vi "UMLEditor Main.vi"(1 "StartProject":string, 3 "StartTarget":string) -> ()   [LabVIEW 2012]
doc: "Main Open UML Modeller VI"
uses:
  <resource>/Framework/Providers/Open_GDS/UML/UMLEditor/UMLEditor ClassToolButtons.ctl
  <resource>/Framework/Providers/Open_GDS/UML/UMLEditor/UMLEditor SequenceToolButtons.ctl
  <resource>/Framework/Providers/Open_GDS/UML/UMLEditor/UMLEditor UseCaseToolButtons.ctl
  <resource>/Framework/Providers/Open_GDS/UML/UMLEditor/UMLEditor StateToolButtons.ctl
  <resource>/Framework/Providers/Open_GDS/UML/UMLEditor/UMLEditor statesType.ctl
  <resource>/Framework/Providers/Open_GDS/UML/UMLEditor/UMLEditor LocalVariablesType.ctl
  <resource>/Framework/Providers/Open_GDS/UML/Graphics_class/Graphics.lvclass
  <resource>/Framework/Providers/Open_GDS/UML/Grid_class/Grid.lvclass
  <resource>/Framework/Providers/Open_GDS/UML/UMLEditor/UMLEditor tooltype.ctl
  <resource>/Framework/Providers/Open_GDS/UML/UMLEditor/UMLEditor toolsType.ctl
  <resource>/Framework/Providers/Open_GDS/UML/Graph_class/private/diagramType.ctl
  <resource>/Framework/Providers/Open_GDS/UML/Graph_class/Graph.lvclass
  <resource>/Framework/Providers/Open_GDS/UML/General/Point/Point Point2D.ctl
  <resource>/Framework/Providers/Open_GDS/UML/General/Rectangle/Rectangle Rectangle2D.ctl
  <resource>/Framework/Providers/Open_GDS/UML/AbstractEdge_class/AbstractEdge.lvclass
  <resource>/Framework/Providers/Open_GDS/UML/UMLEditor/UMLEditor ExportType.ctl
  <resource>/Framework/Providers/Open_GDS/UML/UMLEditor/UMLEditor FlattenCommandType.ctl
  <resource>/Framework/Providers/Open_GDS/UML/UMLEditor/UMLEditor ExecuteCommandType.ctl
  <resource>/Framework/Providers/Open_GDS/UML/ContextHelp/ContextHelp_EventType.ctl
  <resource>/Framework/Providers/Open_GDS/UML/AbstractNode_class/AbstractNode.lvclass
  <resource>/Framework/Providers/Open_GDS/UML/UmlEditor_class/EventData.ctl
  <resource>/Framework/Providers/Open_GDS/UML/UMLEditor/UMLEditor_HotSpotData.ctl
  <resource>/Framework/Providers/Open_GDS/UML/UMLEditor/UMLEditor_HotSpotType.ctl
  <resource>/Framework/Providers/Open_GDS/UML/UMLEditor/UMLEditor_Cursortype.ctl
  <resource>/Framework/Providers/Open_GDS/UML/UMLEditor/UMLEditor MenuActionType.ctl
  <resource>/Framework/Providers/Open_GDS/UML/Graphics_class/LvFontType.ctl
  <resource>/Framework/Providers/Open_GDS/UML/UMLEditor/UMLEditor ToolButtonsAction.ctl
  <resource>/Framework/Providers/Open_GDS/UML/Graphics_class/FontType.ctl
  <resource>/Framework/Providers/Open_GDS/UML/UMLEditor/UMLEditor BusyDialogAction.ctl
  <resource>/Framework/Providers/Open_GDS/UML/UMLEditor/UMLEditor_StoredPathes.ctl
  <resource>/Framework/Providers/Open_GDS/ClassProviders/Common/File/File_StoredPathesActions.ctl
  <resource>/Framework/Providers/Open_GDS/UML/GeneralPathEdge_class/GeneralPathEdge.lvclass
  <vilib>/event_ctls.llb/eventvkey.ctl
  <resource>/Framework/Providers/Open_GDS/UML/ContextHelp/ContextHelp_HelpTexts.ctl
  <resource>/Framework/Providers/Open_GDS/UML/Graph_class/SaveTypes.ctl
  <resource>/Framework/Providers/Open_GDS/UML/ClassNode_class/ClassNode.lvclass
  <resource>/Framework/Providers/Open_GDS/UML/StateDiagramGraph_class/StateDiagramGraph.lvclass
  <resource>/Framework/Providers/Open_GDS/UML/ClassNode_class/ExternalSetTypes.ctl
  <resource>/Framework/Providers/Open_GDS/UML/StateDiagramGraph_class/private/StateDiagramData.ctl
  <resource>/Framework/Providers/Open_GDS/UML/StateDiagramGraph_class/private/ViPathShowOption.ctl
  <resource>/Framework/Providers/Open_GDS/UML/UMLEditor/UMLEditor ClipBoardActionType.ctl
  <resource>/Framework/Providers/Open_GDS/UML/RectangularNode_class/RectangularNode.lvclass
  <resource>/Framework/Providers/Open_GDS/UML/ReversedEngineering/private/ReversedEngineering SyncUmlFromCodeActions.ctl
  <resource>/Framework/Providers/Open_GDS/ClassProviders/Provider_BaseClassInterface/ClassReader_class/ClassReader.lvclass
  <resource>/Framework/Providers/Open_GDS/ClassProviders/Common/CommonVIs/CommonVIs_StereoType.ctl
  <vilib>/Utility/cursorutil.llb/Set Cursor (Icon Pict).vi
  <vilib>/Utility/cursorutil.llb/Set Cursor (Cursor ID).vi
  Instance           2 22Saved   UMLEditor Main .vi
  Instance           1 22Saved   UMLEditor Main .vi
  <resource>/Framework/Providers/Open_GDS/UML/ClassDiagramGraph_class/ClassDiagramGraph.lvclass
  <resource>/Framework/Providers/Open_GDS/UML/SequenceDiagramGraph_class/SequenceDiagramGraph.lvclass
  <resource>/Framework/Providers/Open_GDS/UML/UseCaseDiagramGraph_class/UseCaseDiagramGraph.lvclass
  <resource>/Framework/Providers/Open_GDS/UML/UmlEditor_class/UmlEditor.lvclass
panel:
  out "SearchString":string caption="Search"
  in  "open":bool
  in  "close":bool
  in  "Diagram":u16(ring) items=["State diagram: State1.uml *"]
  out "toolTab":enum32{"Class", "Sequence", "UseCase", "State"}(tab)
  in  "classDiagramTools":T1={"select"=TRUE, "class"=FALSE, "interface"=FALSE, "package"=FALSE, "dependancy"=FALSE, "inheritance"=FALSE, "interfaceImp"=FALSE, "association"=FALSE, "aggregetion"=FALSE, "compAggregetion"=FALSE, "note"=FALSE, "noteConnect"=FALSE}
  in  "sequenceDiagramTools":T2={"select"=TRUE, "Object"=FALSE, "ActionBar"=FALSE, "Call"=FALSE, "note"=FALSE, "noteConnect"=FALSE}
  in  "usecaseDiagramTools":T3={"select"=TRUE, "System"=FALSE, "Actor"=FALSE, "UseCase"=FALSE, "Association"=FALSE, "Generalisation"=FALSE, "Includes"=FALSE, "Extends"=FALSE, "Note"=FALSE, "noteConnect"=FALSE}
  in  "stateDiagramTools":T4={"select"=TRUE, "State"=FALSE, "InitialState"=FALSE, "FinalState"=FALSE, "choice"=FALSE, "StateTransation"=FALSE, "note"=FALSE, "noteConnect"=FALSE}
  out "ProductPicture":picture
  out "Time":i32=21
  out "PictureMenuEvent":string
  out "RevHistory":bool
  in  "Help":bool
  in  "DragAndDropPath":path
  in  "ClassAggregationDialog":T5
  out "Picture":picture
  out "error out":errorcluster
  in  "Project":u16(ring) items=["Open_GDS.lvproj"]
  in  "Help":bool=TRUE
  in  "Case Constant\n(See Context Help) 2":bool
  in  "Target":u16(ring) items=["My Computer"]
  out "StatusBar":string
  in  "Sync":bool
  # "Class aggregation"
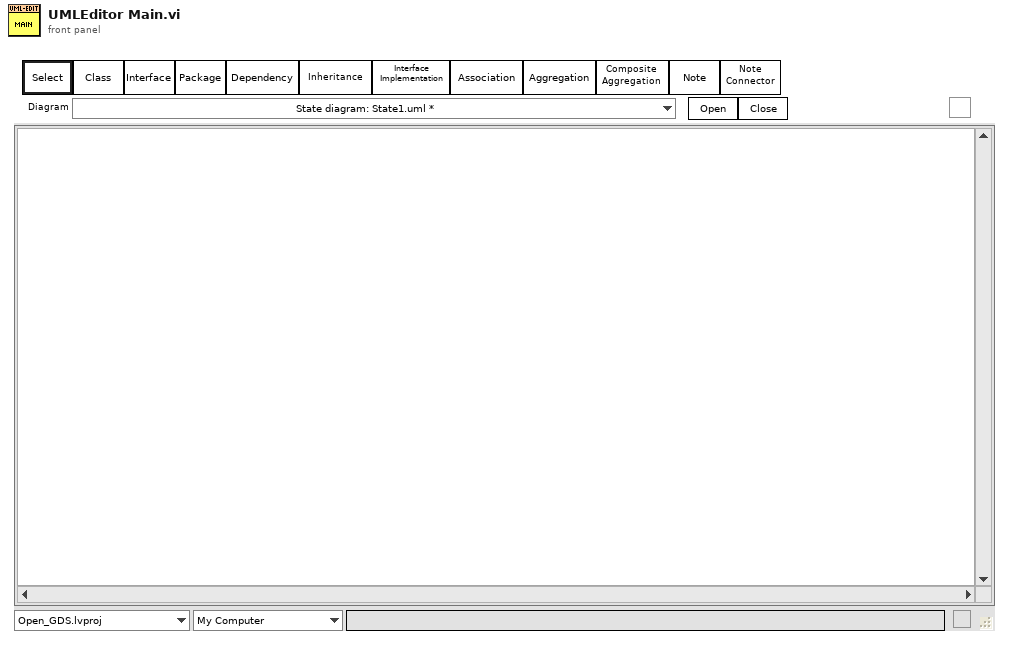
[diagram p1: front panel]
types:
  T1 = typedef "UMLEditor ClassToolButtons.ctl" = cluster{"select":bool, "class":bool, "interface":bool, "package":bool, "dependancy":bool, "inheritance":bool, "interfaceImp":bool, "association":bool, "aggregetion":bool, "compAggregetion":bool, "note":bool, "noteConnect":bool}
  T2 = typedef "UMLEditor SequenceToolButtons.ctl" = cluster{"select":bool, "Object":bool, "ActionBar":bool, "Call":bool, "note":bool, "noteConnect":bool}
  T3 = typedef "UMLEditor UseCaseToolButtons.ctl" = cluster{"select":bool, "System":bool, "Actor":bool, "UseCase":bool, "Association":bool, "Generalisation":bool, "Includes":bool, "Extends":bool, "Note":bool, "noteConnect":bool}
  T4 = typedef "UMLEditor StateToolButtons.ctl" = cluster{"select":bool, "State":bool, "InitialState":bool, "FinalState":bool, "choice":bool, "StateTransation":bool, "note":bool, "noteConnect":bool}
  T5 = cluster{"AddAttribute":bool, "Don'tAddAttribute":bool, "Close":bool, "Text":string}
  T6 = typedef "UMLEditor_Cursortype.ctl" = enum16{"NS", "WE", "NESW", "NWSE"}
  T7 = typedef "UMLEditor LocalVariablesType.ctl" = cluster{"state":T8, "graphics":refnum<class "Graphics.lvclass">, "grid":refnum<class "Grid.lvclass">, "toolType":T9, "tool":T10, "diagramIndex":i32, "diagrams":cluster{"name":string, "diagramType":T11, "unsaved":bool, "graph":refnum<class "Graph.lvclass">, "saveDir":path}[], "zoom":dbl, "hideGrid":bool, "lastMousePoint":T12, "rubberBandStart":T12, "dragStartPoint":T12, "dragStartBounds":T13, "gridColor":u32, "gridSize":dbl, "CONNECT_THRESHOLD":i32, "selcted":T9, "selectedEdge":refnum<class "AbstractEdge.lvclass">, "butDwn":bool, "lastPress":u32, "modified":bool, "offset":T12, "menu":refnum<k9>, "file":path, "saveAs":bool, "newSelected":bool, "exportype":T14, "quit":bool, "revHistory":cluster{"rev":string, "text":string}[], "FlattenCommandSettings":T15, "PopUpMessageEvent":T17, "ResizePanelInProgress":bool, "NodesBounds":T13, "ToolHelp":bool, "ViRef":refnum<vi>, "FP_CtrlEnterEvents":refnum<event-registration>, "SelectedNodes":refnum<class "AbstractNode.lvclass">[], "mouse":refnum<k1>, "RevPlugInPath":path, "Event":refnum<event-registration>, "Action":string, "KeyPressTime":u32, "Cursors":refnum<k1>[], "ObjectHotspots":T18[], "HotSpotCursor":bool, "HotSpotFunction":T19, "Don'tDeleteChildren":bool, "ShiftDown":bool, "CtrlDown":bool, "HotSpotNode":refnum<class "AbstractNode.lvclass">, "Sync":bool, "SyncTime":u32, "ForceSyncNow":bool, "LastSync":timestamp, "XMI_Import":bool}
  T8 = typedef "UMLEditor statesType.ctl" = enum16{"Idle", "CheckLicense", "revHistory", "Init", "Init2", "EditSelected", "RemoveSelected", "PaintComponent", "ChangeZoom", "ChangeGridSize", "Open", "Close", "Save", "ExportPicture", "Export", "Repaint", "Error", "Exit", "QUIT", "CreateScript", "ExecuteScript", "ClassReversedEngineering", "PlugInReverseEngineering", "StateReversedEngineering", "AutoPlace", "ExecuteCommand", "OpenClass", "SyncAll", "StraightenAssociation", "Copy", "Paste", "AddNodeFromProjectTree", "AddNodeFromProjectTree+SyncAll", "PanAndRepaint", "Init3", "CopyPaste", "ApplyDesignPattern", "AnalyseViInStateDiagram", "AutoSync"}
  T9 = typedef "UMLEditor tooltype.ctl" = enum16{"None", "Node", "Edge"}
  T10 = typedef "UMLEditor toolsType.ctl" = enum16{"CD_Select", "CD_Class", "CD_Interface", "CD_Package", "CD_Note", "CD_Dependency", "CD_Inheritance", "CD_InterfaceImp", "CD_Association", "CD_Aggregation", "CD_Composite", "CD_NoteConn", "SQD_Select", "SQD_Object", "SQD_ActionBar", "SQD_Note", "SQD_Call", "SQD_NoteConn", "UD_Select", "UD_System", "UD_Actor", "UD_UseCase", "UD_Note", "UD_Assoiciation", "UD_Generalization", "UD_GeneralizationIncludes", "UD_GeneralizationExtends", "UD_Realization", "UD_Relationship", "UD_NoteEdge", "STD_Select", "STD_State", "STD_InitailState", "STD_FinalState", "STD_ChoiseState", "STD_StateTransation", "STD_Note", "STD_NoteEdge"}
  T11 = typedef "Graph.lvclass/diagramType.ctl" = enum16{"None", "Class", "Sequency", "State", "UseCase"}
  T12 = typedef "Point Point2D.ctl" = cluster{"x":dbl, "y":dbl}
  T13 = typedef "Rectangle Rectangle2D.ctl" = cluster{"x":dbl, "y":dbl, "width":dbl, "height":dbl}
  T14 = typedef "UMLEditor ExportType.ctl" = enum16{"None", "Printer", "png", "jpg", "roseUML"}
  T15 = typedef "UMLEditor FlattenCommandType.ctl" = cluster{"Command":T16, "CommandData":variant}
  T16 = typedef "UMLEditor ExecuteCommandType.ctl" = enum16{"SyncUmlFromCode", "SyncCodeFromUML", "OpenClass", "OpenFile", "CreateClass", "CreateVI", "OpenClassAttribute", "LocateInProject"}
  T17 = typedef "ContextHelp_EventType.ctl" = refnum<user-event>
  T18 = typedef "UMLEditor_HotSpotData.ctl" = cluster{"Node":refnum<class "AbstractNode.lvclass">, "HotSpot":T12, "Function":T19}
  T19 = typedef "UMLEditor_HotSpotType.ctl" = enum16{"N", "NE", "E", "SE", "S", "SW", "W", "NW", "Expand", "Collaps"}
  T20 = typedef "UMLEditor MenuActionType.ctl" = enum16{"EnableSave", "EnablePaste", "DisablePaste", "DiableSave", "AddRecentFile", "disablePropDel", "enablePropDel", "enablePropDisDel", "diasbleClassRel", "enableClassRel", "Class", "State", "Other", "EnableXMI", "DisableXMI"}
  T21 = typedef "Graphics.lvclass/FontType.ctl" = cluster{"Font Name:":string, "Size":i16, "Strikeout?":bool, "Italic?":bool, "Underline?":bool, "Outline?":bool, "Shadow?":bool, "Bold?":bool}
  T22 = enum16{"CreateAggregation", "DeleteAggregation", "SetReferneces", "HideCluster", "GetStatus"}
  T23 = typedef "UMLEditor ToolButtonsAction.ctl" = enum16{"SelectSelect", "SetReferneces"}
  T24 = typedef "Graphics.lvclass/LvFontType.ctl" = enum16{"User-specified Font", "Application Font", "System Font", "Dialog Font"}
  T25 = typedef "UMLEditor_StoredPathes.ctl" = enum16{"LastSearchPath", "QueuedArrayStateVI", "ClassBasePath", "ViTemplatePath", "ApplicationTemplatePath", "IniFilePath", "WizDir", "RevPlugInPath"}
  T26 = typedef "UMLEditor BusyDialogAction.ctl" = enum16{"Initialize", "Open(VIs)", "Open(i)", "Send_I-Value", "SendStatusMessage", "GetBusyDialogStatus", "Close", "Quit"}
  T27 = enum16{"SetPopUpEventTask", "GetStatus", "SetOpenState", "SetDialogCaller", "SetToolHelp"}
  T28 = typedef "File_StoredPathesActions.ctl" = enum16{"Get Path", "Set Path", "Delete Path", "Clear All Paths"}
  T29 = typedef "ContextHelp_HelpTexts.ctl" = enum16{"None(Hide)", "Default", "Help", "Welcome", "GettingStarted", "ClassDiagram_Help", "SequenceDiagram_Help", "UseCaseDiagram_Help", "BSelect", "BClass", "BInterface", "BPackage", "BNote", "BDependency", "BInheritance", "BInterfaceImplementation", "BAssociation", "BAggregation", "BCompAggregation", "BNoteConnector", "BObject", "BActionBar", "BCall", "BSystem", "BActor", "BUseCase", "BGeneralization", "BIncludes", "BExtends", "BUseCaseDiagramAssociation", "ClassRelationshipEdge editDialog_Bent Style", "ClassRelationshipEdge editDialog_RelationType", "ClassRelationshipEdge editDialog_Reverse association", "ClassRelationshipEdge editDialog_Start label", "ClassRelationshipEdge editDialog_Middle label", "ClassRelationshipEdge editDialog_End label", "UMLEditor reversedEngineering_Pathes", "ReversedEngineering StateReverseDialog_Help", "ReversedEngineering StateQueuedSettings_Help", "UMLEditor reversedEngineering_AddTopVIs", "UMLEditor reversedEngineering_AddClasses", "UMLEditor reversedEngineering_AddDirs", "UMLEditor reversedEngineering_Recursively", "UMLEditor reversedEngineering_Remove", "UMLEditor reversedEngineering_ClearList", "UMLEditor reversedEngineering_HideSubAss", "UMLEditor reversedEngineering_CreateTypes", "UMLEditor reversedEngineering_OnlyInheritance", "UMLEditor reversedEngineering_CreateApplication", "UMLEditor reversedEngineering_OK", "UMLEditor reversedEngineering_Cancel", "UMLEditor reversedEngineering_Help", "UMLEditor createWizardScriptFile_ScriptfilePath", "UMLEditor createWizardScriptFile_ClassPath", "UMLEditor createWizardScriptFile_Use", "UMLEditor createWizardScriptFile_PrivateDirName", "UMLEditor createWizardScriptFile_DirAppend", "UMLEditor createWizardScriptFile_Separator Character", "UMLEditor createWizardScriptFile_OK", "UMLEditor createWizardScriptFile_Cancel", "UMLEditor createWizardScriptFile_Help", "ClassNode editDialog_Class Name", "InterfaceNode editDialog_Class Name", "ClassNode editDialog_Attribute", "ClassNode editDialog_Methods", "InterfaceNode editDialog_Methods", "ClassNode editDialog_connection", "InterfaceNode editDialog_connection", "ClassNode editDialog_StereoType", "ClassNode editDialog_ShowAttrib", "ClassNode editDialog_ShowMethods", "ClassNode editDialog_ClassPath", "ClassNode editDialog_AddAttribute", "ClassNode editDialog_AddMethod", "InterfaceNode editDialog_AddMethod", "ClassNode AttributeGuide_AttributeName", "ClassNode AttributeGuide_Array?", "ClassNode AttributeGuide_Data Type", "ClassNode AttributeGuide_RefName", "ClassNode AttributeGuide_Preview", "ClassNode AttributeGuide_OK", "ClassNode AttributeGuide_Cancel", "ClassNode MethodGuide_Visibility", "ClassNode MethodGuide_Method Name", "ClassNode MethodGuide_Preview", "ClassNode MethodGuide_OK", "ClassNode MethodGuide_Cancel", "CallNode EditCallProperties_AllButtons", "ObjectNode EditObjectlProperties_AllButtons", "ActorNode EditActorProperties_AllButtons", "UseCaseRelationshipNode EditUseCaselProperties_AllButtons", "UseCaseNode EditUseCaselProperties_AllButtons", "SystemNode EditSystemProperties_AllButtons", "ReversedEngineering UpdateAttributes_AllButtons", "StateNode editDialog_AllButtons", "StateTransition editDialog_AllButtons", "ArrangeNodes Main_Picture", "ArrangeNodes Main_Zoom", "ArrangeNodes Main_Auto Zoom", "ArrangeNodes Main_shorten", "ArrangeNodes Main_Min Length", "ArrangeNodes Main_Max Length", "ArrangeNodes Main_increase", "ArrangeNodes Main_decrease", "ArrangeNodes Main_Shake", "ArrangeNodes Main", "BState", "BInitialState", "BFinalState", "BStateTransition", "StateDiagram_Help", "StateDiagram_PropertiesAllButtons", "ReversedEngineering StateReverseDialog_ClearStates", "ReversedEngineering StateReverseDialog_UseQueuedStateMachines", "ReversedEngineering StateReverseDialog_QueuedSettings", "ReversedEngineering StateReverseDialog_SearchForVIs", "ReversedEngineering StateReverseDialog_SearchCriteria", "OptionsDialog_ClassBasePath", "OptionsDialog_VIPath", "OptionsDialog_ApplicationPath", "OptionsDialog_WizDir", "OptionsDialog_IniFilePath", "OptionsDialog_DefineColors", "OptionsDialog_Help", "OptionsDialog_CreateTypes", "ClassRelationshipEdge editDialog_SplitWire"}
  T30 = typedef "Graph.lvclass/SaveTypes.ctl" = enum16{"Normal", "XMI"}
  T31 = typedef "ClassNode.lvclass/ExternalSetTypes.ctl" = enum16{"Name", "Attributes", "Methods", "Position", "ShowMethods", "ShowAttributes", "ClassPath"}
  T32 = typedef "StateDiagramGraph.lvclass/StateDiagramData.ctl" = cluster{"VI-Path":path, "ShowOption":T33}
  T33 = typedef "StateDiagramGraph.lvclass/ViPathShowOption.ctl" = enum16{"Don't Show", "Show Relative Path", "Show Absolute Path"}
  T34 = typedef "UMLEditor ClipBoardActionType.ctl" = enum16{"Init", "EmptyClipBoard", "InsertToClipBoard", "PasteContentAtPos"}
  T35 = enum16{"Left Button", "Center Button", "Right Button", "Window Close"}
  T36 = typedef "ReversedEngineering SyncUmlFromCodeActions.ctl" = enum16{"GetAttributes&MethodsFromCode", "GetAll"}
  T37 = typedef "CommonVIs_StereoType.ctl" = enum16{"None", "TYPE", "ENUM", "ABSTRACT", "ACTOR", "GUI", "SINGLETON", "SIGNAL", "BOUNDARY", "ENTITY", "CONTROL", "LEGACY", "APPLICATION", "VI", "LVLIB"}
  T38 = enum8{"Enabled", "Disabled", "Disabled and Grayed Out"}
  T39 = cluster{"name":string, "diagramType":T11, "unsaved":bool, "graph":refnum<class "Graph.lvclass">, "saveDir":path}[]
  T40 = cluster{"name":string, "diagramType":T11, "unsaved":bool, "graph":refnum<class "Graph.lvclass">, "saveDir":path}
  T41 = typedef "eventsource.ctl" = u32
  T42 = typedef "LVMouseTypeDef.ctl" = cluster{"Mouse Position":cluster{"X":i32, "Y":i32}, "Mouse Modifiers":cluster{"Button Down":bool, "Shift Mod":bool, "Menu Mod":bool, "Option Mod":bool}}
  T43 = typedef "LVBoundsTypeDef.ctl" = cluster{"Width":u32, "Height":u32}
  T44 = typedef "LVPointTypeDef.ctl" = cluster{"Horizontal":i16, "Vertical":i16}
  T45 = typedef "UMLEditor EditorActionType.ctl" = enum16{"NoAction", "Repaint", "ExecuteCommand"}
  T46 = typedef "LVPoint32TypeDef.ctl" = cluster{"Horizontal":i32, "Vertical":i32}
  T47 = cluster{"[0]":bool, "[1]":bool, "[2]":bool, "[3]":bool, "[4]":bool, "[5]":bool, "[6]":bool, "[7]":bool, "[8]":bool, "[9]":bool, "[10]":bool, "[11]":bool}
  T48 = cluster{"[0]":bool, "[1]":bool, "[2]":bool, "[3]":bool, "[4]":bool, "[5]":bool, "[6]":bool, "[7]":bool, "[8]":bool, "[9]":bool}
  T49 = cluster{"[0]":bool, "[1]":bool, "[2]":bool, "[3]":bool, "[4]":bool, "[5]":bool, "[6]":bool, "[7]":bool}
  T50 = cluster{"[0]":bool, "[1]":bool, "[2]":bool, "[3]":bool, "[4]":bool, "[5]":bool}
  T51 = cluster{"button 1":bool, "button 2":bool, "button 3":bool, "button 4":bool}
  T52 = cluster{"Horizontal":i32, "Vertical":i32, "Scrolling":i32}
  T53 = typedef "LVRectTypeDef.ctl" = cluster{"Left":i16, "Top":i16, "Right":i16, "Bottom":i16}
  T54 = typedef "eventvkey.ctl" = enum16{"ASCII", "Enter", "Return", "Shift", "Ctrl", "Alt", "Cmd", "Opt", "Caps", "NumLock", "Clear", "Break", "Up", "Down", "Left", "Right", "Insert", "Delete", "Home", "End", "PageUp", "PageDown", "Escape", "Help", "Pause", "ScrollLock", "F1", "F2", "F3", "F4", "F5", "F6", "F7", "F8", "F9", "F10", "F11", "F12", "F13", "F14", "F15", "F16", "F17", "F18", "F19", "F20", "F21", "F22", "F23", "F24", "Play", "VolumeUp", "VolumeDown", "Mute", "Two Byte Char"}
  T55 = typedef "lveventtype.ctl" = enum32{"Null", "Timeout", "Annotation Menu Selection", "Annotation Menu Selection?", "App Instance Close", "App Instance Close?", "Autoscale Range Change", "Cell Edit", "Cell Edit?", "Cursor Grab", "Cursor Grab?", "Cursor Menu Selection", "Cursor Menu Selection?", "Cursor Move", "Cursor Release", "Data Change", "Direction Change", "Display State Change", "Drag Ended", "Drag Enter", "Drag Leave", "Drag Over", "Drag Source Update", "Drag Starting", "Drag Starting?", "Drop", "Exec State Change", "Key Down", "Key Down?", "Key Repeat", "Key Repeat?", "Key Up", "Listbox Double Click", "Menu Activation?", "Menu Selection (App)", "Menu Selection? (App)", "Menu Selection (User)", "Mouse Down", "Mouse Down?", "Mouse Enter", "Mouse Leave", "Mouse Move", "Mouse Up", "NI Security User Change (App)", "Pane Size", "Panel Close", "Panel Close?", "Panel Resize", "Plot Attribute Change", "Scale Range Change", "Shortcut Menu Activation?", "Shortcut Menu Selection (App)", "Shortcut Menu Selection? (App)", "Shortcut Menu Selection (User)", "Tree Double Click", "Tree Drag", "Tree Drag?", "Tree Drop", "Tree Drop?", "Tree Item Close", "Tree Item Close?", "Tree Item Open", "Tree Item Open?", "Value Change"}
  T56 = cluster{"Shift":bool, "Ctrl":bool, "Alt":bool, "Cmd":bool, "Opt":bool}
  T57 = typedef "ContextHelp_ShowType.ctl" = cluster{"Header":string, "Picture":picture, "Text":string}
  T58 = enum32{"existing file", "new file", "new or existing file", "existing dir", "new dir", "new or existing dir", "existing file (use LLBs)", "new file (use LLBs)", "new or existing file (use LLBs)", "new or existing file or directory (use LLBs)"}
  T59 = cluster{"startNode":refnum<class "AbstractNode.lvclass">, "endNode":refnum<class "AbstractNode.lvclass">}
  T60 = enum32{"Invalid", "Standard", "Closed", "Hidden", "Minimized", "Maximized"}
  T61 = typedef "AbstractNode.lvclass/NodeConnectionStatsType.ctl" = enum16{"NA", "Connect", "DisConnect"}
  T62 = typedef "Librarian File Info Out.ctl" = cluster{"creation date":u32, "last mod date":u32, "type":string, "creator":string, "LV version":i32, "size":i32, "top level":bool}
  T63 = typedef "DesignPatterns_Node.ctl" = cluster{"ID":string, "Type":T64, "Name":string, "Stereotype":string, "X":i32, "Y":i32, "TypeSpecificData":variant}
  T64 = typedef "DesignPatterns_NodeType.ctl" = enum16{"Class", "Interface", "Note", "Package"}
  T65 = typedef "DesignPatterns_Link.ctl" = cluster{"ID":string, "Type":T66, "Name":string, "StartText":string, "EndText":string, "From":string, "To":string}
  T66 = typedef "DesignPatterns_LinkType.ctl" = enum16{"Dependency", "Inheritance", "Interface", "Association", "Aggregation", "CompositeAggregation"}
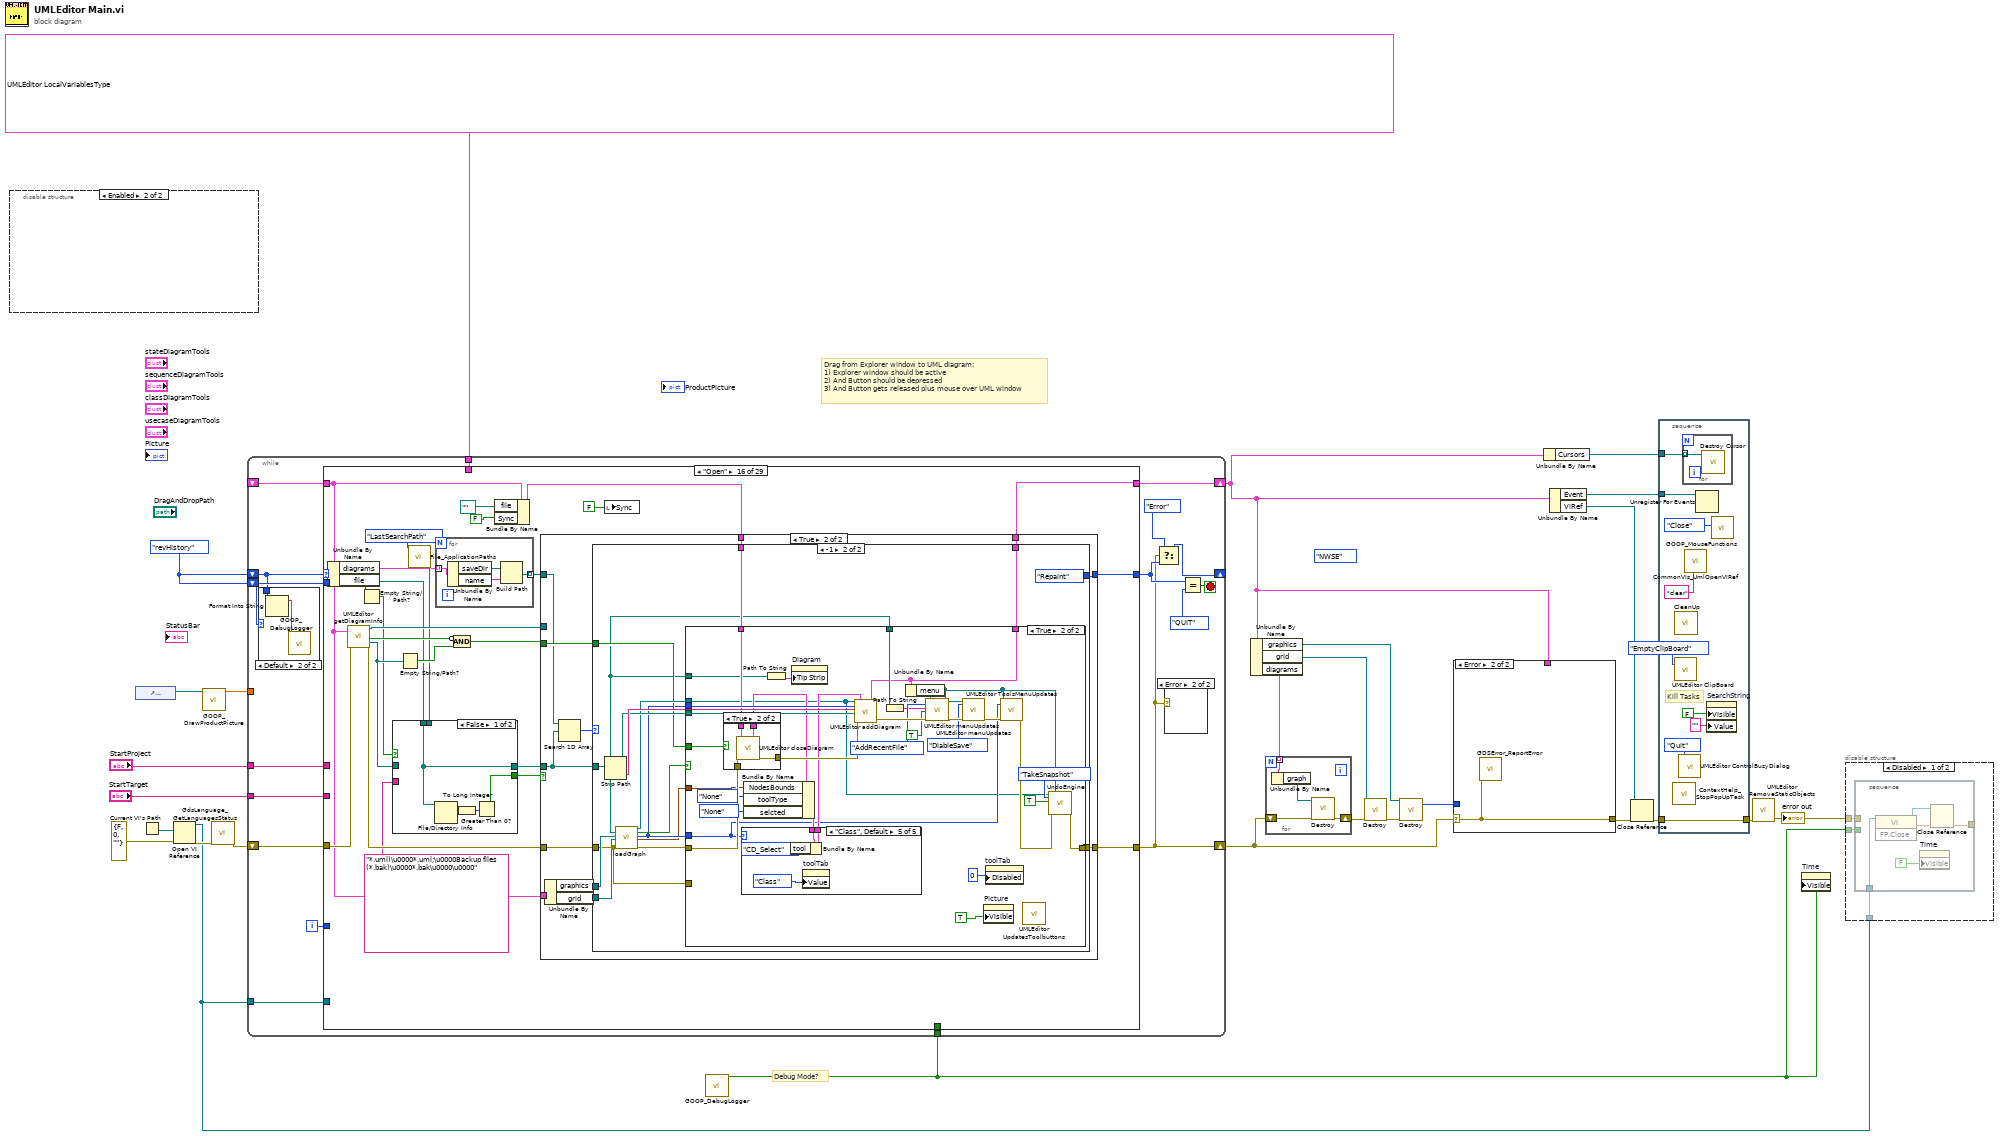
[diagram p0: block diagram]
diagram:
  (unwired) UMLEditor_Cursortype."NWSE" ("CursorType")
  w21 = UMLEditor_statesType."revHistory" ("state")
  # "Debug Mode?"
  # "Drag from Explorer window to UML diagram:\n1) Explorer window should be active\n2) And Button should be depressed\n3) And Button gets released plus mouse over UML window"
  n1 = disable-structure shown="Enabled" {
    frame Disabled {
      n2 = local write "ClassAggregationDialog"(T5 {"AddAttribute"=FALSE, "Don'tAddAttribute"=FALSE, "Close"=FALSE, "Text"="A class that aggregates\nanother class, should have\na reference to that class\nin its attribute.\n\nDo you want to automatically\nadd this attribute?"} ("ClassAggregationDialog")) -> ()
    }
    frame Enabled {
    }
  }
  n3 = control-ref of="ProductPicture"() -> (w3:refnum<vi>)
  n4 = Current VI's Path() -> (path=w14:path)
  n5 = Open VI Reference(vi path=w14, error in (no error)=errorcluster {"status"=FALSE, "code"=0, "source"=""} ("error out")) -> (vi reference=w7:refnum<vi>, error out=w11:errorcluster)  [unwired: 4 out]
  n6 = call <resource>:"GOOP_DrawProductPicture.vi"("ProductPictureControl"=w3) -> ("Zoom Factor"=w2:sgl)  [unwired: 10 in]
  n7 = call <resource>:"GdsLanguage_GetLanguagesStatus.vi"("error in (no error)"=w11) -> ("error out"=w10:errorcluster)  [unwired: 18 out]
  n8 = call <resource>:"GOOP_DebugLogger.vi"() -> ("Debugging"=w1:bool)  [unwired: 10 in, 1 out]
  n9 = while {
    shift-right: [w38] -> _
    shift-left: w21 -> [w29]
    shift-right: [w32] -> w5
    shift-left: w10 -> [w43]
    shift-right: [w40] -> w9
    shift-left: _ -> [w39]
    tunnel: T7 {"state"=enum."Idle", "graphics"=refnum, "grid"=refnum, "toolType"=enum."None", "tool"=enum."CD_Select", "diagramIndex"=0, "diagrams"=[], "zoom"=0.0, "hideGrid"=FALSE, "lastMousePoint"={"x"=0.0, "y"=0.0}, "rubberBandStart"={"x"=0.0, "y"=0.0}, "dragStartPoint"={"x"=0.0, "y"=0.0}, "dragStartBounds"={"x"=0.0, "y"=0.0, "width"=0.0, "height"=0.0}, "gridColor"=0, "gridSize"=0.0, "CONNECT_THRESHOLD"=0, "selcted"=enum."None", "selectedEdge"=refnum, "butDwn"=FALSE, "lastPress"=0, "modified"=FALSE, "offset"={"x"=0.0, "y"=0.0}, "menu"=refnum, "file"=path "", "saveAs"=FALSE, "newSelected"=FALSE, "exportype"=enum."None", "quit"=FALSE, "revHistory"=[], "FlattenCommandSettings"={"Command"=enum."SyncUmlFromCode", "CommandData"=variant}, "PopUpMessageEvent"=refnum, "ResizePanelInProgress"=FALSE, "NodesBounds"={"x"=0.0, "y"=0.0, "width"=0.0, "height"=0.0}, "ToolHelp"=FALSE, "ViRef"=refnum, "FP_CtrlEnterEvents"=refnum, "SelectedNodes"=[], "mouse"=refnum, "RevPlugInPath"=path "", "Event"=refnum, "Action"="", "KeyPressTime"=0, "Cursors"=[], "ObjectHotspots"=[], "HotSpotCursor"=FALSE, "HotSpotFunction"=enum."N", "Don'tDeleteChildren"=FALSE, "ShiftDown"=FALSE, "CtrlDown"=FALSE, "HotSpotNode"=refnum, "Sync"=FALSE, "SyncTime"=0, "ForceSyncNow"=FALSE, "LastSync"=timestamp(0 s since 1904-01-01), "XMI_Import"=FALSE} ("localVariables") -> [w41]
    shift-left: w21 -> [w36]
    tunnel: "StartProject" -> [w34]
    tunnel: w1 -> [w33]
    tunnel: w7 -> [w31]
    tunnel: "StartTarget" -> [w30]
    tunnel: w2 -> [_]
    i -> [w35]
    stop <- w45 stop-if-true
    n10 = case shown="Default" w29 {
      tunnel: w29 -> [_ w47]
      frame "Idle", "PaintComponent", "Repaint" {
      }
      frame Default {
        n11 = Format Into String(w47) -> (resulting string=w46:string)  [unwired: 3 in, 1 out]
        n12 = call <resource>:"GOOP_DebugLogger.vi"("State"=w46) -> ()  [unwired: 9 in, 2 out]
      }
    }
    n13 = case shown="\"Open\"" w29 {
      selector: w29 -> [_ _ _ _ _ w276 _ w3910 _ w4191 _ _ _ _ _ _ _ w4874 w4909 _ _ _ _ _ _ _ _ _ _]
      tunnel: [UMLEditor_statesType."CheckLicense" ("state") w55 UMLEditor_statesType."Init2" ("state") UMLEditor_statesType."Init3" ("state") w231 w269 w3825 w3921 w4117 w4198 UMLEditor_statesType."Repaint" ("state") UMLEditor_statesType."Idle" ("state") UMLEditor_statesType."Repaint" ("state") UMLEditor_statesType."Repaint" ("state") w4531 w4636 w4771 UMLEditor_statesType."Repaint" ("state") w4910 UMLEditor_statesType."Repaint" ("state") w5088 UMLEditor_statesType."Idle" ("state") UMLEditor_statesType."Repaint" ("state") w5319 UMLEditor_statesType."Repaint" ("state") UMLEditor_statesType."Repaint" ("state") UMLEditor_statesType."Repaint" ("state") w5758 w5789] -> w37
      tunnel: w43 -> [w49 w54 w88 w202 w246 w281 w3824 w3930 w4109 w4195 w4219 w4289 w4340 w4474 w4550 w4651 w4775 w4880 w4916 w5055 w5092 w5150 w5296 w5315 w5600 w5655 w5735 w5745 w5779]
      tunnel: [w49 w58 w112 w187 w245 w282 w3824 w3923 w4119 w4194 w4223 w4280 w4342 w4467 w4549 w4646 w4777 w4879 w4915 w5044 w5076 w5119 w5295 w5318 w5601 w5643 w5723 w5759 w5785] -> w32
      tunnel: w41 -> [w52 _ _ _ _ _ _ _ _ _ _ _ _ _ _ _ _ _ _ _ _ _ _ _ _ _ _ _ _]
      tunnel: [w51 w53 w94 w207 w244 w278 w3820 w3924 w4118 w4192 w4214 w4260 w4336 w4464 w4545 w4641 w4770 w4876 w4912 w5060 w5079 w5125 w5293 w5312 w5599 w5646 w5731 w5752 w5780] -> w40
      tunnel: w39 -> [_ w53 w114 w183 w236 w272 w3809 w3915 w4105 w4192 w4215 w4260 w4332 w4470 w4528 w4634 w4767 w4877 w4906 w5060 w5079 w5129 w5294 w5309 w5598 w5632 w5727 w5751 w5780]
      tunnel: w36 -> [_ w63 _ _ _ _ _ _ _ _ _ _ _ _ w4534 _ w4769 w4878 _ _ _ w5141 _ _ _ w5637 _ _ w5782]
      tunnel: w35 -> [_ _ _ _ _ _ _ _ _ _ _ _ _ _ _ _ _ _ _ _ _ _ _ _ _ _ _ _ _]
      tunnel: w34 -> [_ _ _ w195 _ _ _ _ _ _ _ _ _ _ _ _ _ _ _ _ _ _ _ _ _ _ _ _ _]
      tunnel: w33 -> [_ _ _ _ _ _ _ _ _ _ _ _ _ _ _ _ _ _ _ _ _ w5118 _ _ _ _ _ _ _]
      tunnel: w31 -> [_ _ _ _ _ w271 _ _ _ _ _ _ _ _ _ _ _ _ _ _ _ _ _ _ _ _ _ _ _]
      tunnel: w30 -> [_ _ _ w174 _ _ _ _ _ _ _ _ _ _ _ _ _ _ _ _ _ _ _ _ _ _ _ _ _]
      frame "revHistory" {
        n14 = Bundle By Name(cluster=w52, "revHistory"=cluster{"rev":string, "text":string}[] []) -> (w51:T7)
      }
      frame "CheckLicense" {
        n15 = Equal?(x=w63, y=UMLEditor_statesType."Idle" ("state")) -> (x = y?=w59:bool)
        n16 = Current VI's Menubar() -> (w57:refnum<k9>)
        n17 = call <resource>:"UMLEditor menuUpdates.vi"("menu"=w57, "menuAction"=UMLEditor_MenuActionType."EnableXMI", "error in (no error)"=w54) -> ("error out"=w58:errorcluster)  [unwired: 3 in, 13 out]
        n18 = Select(t=UMLEditor_statesType."Idle" ("state"), s=w59, f=UMLEditor_statesType."Init" ("state")) -> (s? t:f=w55:T8)
      }
      frame "Init" {
        w137 = T12 {"x"=nan, "y"=nan} ("lastMousePoint")
        w75 = 10.0  # gridSize
        w111 = 0 ("offsetX")
        w65 = FALSE ("Help")
        w113 = "Untitled 1" ("name")
        w76 = u32 14803425
        n19 = control-ref of="Picture"() -> (w73:refnum<vi>)
        n20 = call <resource>:"Init.vi"("error in (no error)"=w88) -> ("Event"=w87:refnum<user-event>, "error out"=w86:errorcluster)  [unwired: 17 out]
        n21 = property on="ClassAggregationDialog" class="Clust (strict)"("Visible"=FALSE) -> ()  [unwired: 2 in, 2 out]
        n22 = register-events(error in=w86, w87) -> (reference out=w85:refnum<event-registration>, error out=w67:errorcluster)  [unwired: 1 in]
        n23 = call <resource>:"Graphics_Create.vi"("screenRef"=w73, "error in (no error)"=w67) -> ("reference out"=w129:refnum<class "Graphics.lvclass">, "error out"=w128:errorcluster)  [unwired: 1 in, 15 out]
        n24 = call <resource>:"setFont.vi"("reference"=w129, "fontType"=LvFontType."User-specified Font", "font"=T21 {"Font Name:"="Ariel", "Size"=14, "Strikeout?"=FALSE, "Italic?"=FALSE, "Underline?"=FALSE, "Outline?"=FALSE, "Shadow?"=FALSE, "Bold?"=FALSE}, "error in (no error)"=w128) -> ("reference out"=w127:refnum<class "Graphics.lvclass">, "error out"=w126:errorcluster)  [unwired: 14 out]
        n25 = property on="Picture" class="Pict"("Visible"=TRUE) -> ()  [unwired: 2 in, 2 out]
        n26 = control-ref of="AddAttribute"() -> (w79:refnum<vi>)
        n27 = control-ref of="Don'tAddAttribute"() -> (w78:refnum<vi>)
        n28 = control-ref of="ClassAggregationDialog"() -> (w74:refnum<vi>)
        n29 = control-ref of="Text"() -> (w77:refnum<vi>)
        n30 = call <resource>:"getScreenBounds.vi"("reference"=w127, "error in (no error)"=w126) -> ("reference out"=w144:refnum<class "Graphics.lvclass">, "bounds"=w118:T13, "error out"=w150:errorcluster)  [unwired: 15 out]
        n31 = control-ref of="classDiagramTools"() -> (w109:refnum<vi>)
        n32 = control-ref of="sequenceDiagramTools"() -> (w105:refnum<vi>)
        n33 = control-ref of="usecaseDiagramTools"() -> (w104:refnum<vi>)
        n34 = control-ref of="stateDiagramTools"() -> (w103:refnum<vi>)
        n35 = call <resource>:"Grid_Create.vi"("gridColor"=w76, "error in (no error)"=w150) -> ("reference out"=w147:refnum<class "Grid.lvclass">, "error out"=w148:errorcluster)  [unwired: 2 in, 14 out]
        n36 = call <resource>:"setGrid.vi"("reference"=w147, "gridX"=w75, "gridY"=w75, "error in (no error)"=w148) -> ("reference out"=w146:refnum<class "Grid.lvclass">, "error out"=w149:errorcluster)  [unwired: 14 out]
        n37 = call <resource>:"UMLEditor UpdatesToolbuttons.vi"("ClassTool"=w109, "SequenceTool"=w105, "UseCaseTool"=w104, "StateTool"=w103, "Action(SelectSelect)"=UMLEditor_ToolButtonsAction."SetReferneces") -> ("error out"=w107:errorcluster)  [unwired: 1 in, 13 out]
        n38 = call <resource>:"UMLEditor_AggregationClusterDialogControl.vi"("OK-Button"=w79, "Cancel-Button"=w78, "String"=w77, "Cluster"=w74, "Action(SelectSelect)"=T22."SetReferneces", "screenRef"=w73) -> ()  [unwired: 3 in, 11 out]
        n39 = call-dynamic "draw.vi"("reference"=w146, "graphics"=w144, "bounds"=w118, "error in (no error)"=w149) -> ("reference out"=w145:refnum<class "Grid.lvclass">, "error out"=w100:errorcluster)  [unwired: 14 in]
        n40 = call <resource>:"UMLEditor UpdatesToolbuttons.vi"("error in (no error)"=w107, "Action(SelectSelect)"=UMLEditor_ToolButtonsAction."SelectSelect") -> ()  [unwired: 4 in, 14 out]
        n41 = call <resource>:"updateScreen.vi"("reference"=w144, "error in (no error)"=w100) -> ("reference out"=w143:refnum<class "Graphics.lvclass">, "error out"=w90:errorcluster)  [unwired: 16 out]
        n42 = call <resource>:"UMLEditor_IniFilePath.vi"("error in (no error)"=w90) -> ("Get Path"=w91:path, "error out"=w89:errorcluster)  [unwired: 1 in, 16 out]
        n43 = Current VI's Menubar() -> (w81:refnum<k9>)
        n44 = call <resource>:"UMLEditor loadIniFileInfo.vi"("menu"=w81, "iniFile"=w91, "error in (no error)"=w89) -> ("StabilityProblems"=w64:bool, "SyncTime"=w66:u32, "Ini-FileFound"=w96:bool, "ToolHelp"=w97:bool, "LastDiagramType"=w98:T11, "FileToOpen"=w68:path, "error out"=w99:errorcluster)  [unwired: 10 out]
        n45 = property on="Diagram" class="Ring (strict)"("Tip Strip"=w113) -> ()  [unwired: 2 in, 2 out]
        n46 = case shown="\"Class\", Default" w98 {
          tunnel: [w156 w158 w162 w168] -> w83
          tunnel: [w155 w160 w163 w169] -> w102
          tunnel: [diagramType."Class" ("diagramType") diagramType."Sequency" ("diagramType") diagramType."UseCase" ("diagramType") diagramType."State" ("diagramType")] -> w101
          tunnel: w99 -> [w153 w159 w164 w170]
          tunnel: [enum32{"Class", "Sequence", "UseCase", "State"}."Class" ("toolTab") enum32{"Class", "Sequence", "UseCase", "State"}."Sequence" ("toolTab") enum32{"Class", "Sequence", "UseCase", "State"}."UseCase" ("toolTab") enum32{"Class", "Sequence", "UseCase", "State"}."State" ("toolTab")] -> w95
          frame "Class", Default {
            n47 = call <resource>:"ClassDiagramGraph_Create.vi"("error in (no error)"=w153) -> ("reference out"=w156:refnum<class "ClassDiagramGraph.lvclass">, "error out"=w155:errorcluster)  [unwired: 2 in, 15 out]
          }
          frame "Sequency" {
            n48 = call <resource>:"SequenceDiagramGraph_Create.vi"("error in (no error)"=w159) -> ("reference out"=w158:refnum<class "SequenceDiagramGraph.lvclass">, "error out"=w160:errorcluster)  [unwired: 2 in, 15 out]
          }
          frame "UseCase" {
            n49 = call <resource>:"UseCaseDiagramGraph_Create.vi"("error in (no error)"=w164) -> ("reference out"=w162:refnum<class "UseCaseDiagramGraph.lvclass">, "error out"=w163:errorcluster)  [unwired: 2 in, 15 out]
          }
          frame "State" {
            n50 = call <resource>:"StateDiagramGraph_Create.vi"("error in (no error)"=w170) -> ("reference out"=w168:refnum<class "StateDiagramGraph.lvclass">, "error out"=w169:errorcluster)  [unwired: 3 in, 14 out]
          }
        }
        "toolTab" <- w95
        n51 = case shown="True" w96 {
          frame False {
            n52 = call <resource>:"UMLEditor GettingStartedDialog.vi"() -> ()  [unwired: 1 out]
          }
          frame True {
          }
        }
        n53 = Unbundle By Name(w114) -> ("diagrams"=w133:T39)
        n54 = call <resource>:"UMLEditor ToolsMenuUpdates.vi"("menu"=w81, "diagramType"=w101, "error in (no error)"=w102) -> ("error out"=w93:errorcluster)  [unwired: 1 in, 15 out]
        n55 = Index Array(array=w133) -> (element=w132:T40)  [unwired: 1 in]
        n56 = Bundle By Name(cluster=w132, "name"=w113, "diagramType"=w101, "unsaved"=FALSE, "graph"=w83, "saveDir"=path "") -> (w120:T40)
        n57 = local write "Help"(w65) -> ()
        n58 = property on="SearchString" class="Str"("Visible"=FALSE, "Value"="" ("SearchString")) -> ()  [unwired: 2 in, 2 out]
        n59 = call <resource>:"GOOP_MouseFunctions.vi"("error in (no error)"=w93, "StabilityProblem"=w64, "Action(Read)"=enum16{"Init", "Read", "Close"}."Init") -> ("error out"=w92:errorcluster)  [unwired: 6 in, 2 out]
        n60 = Build Array(w120) -> (w130:T39)
        n61 = Set Menu Item Info(7:"Undo" ("item tag"), 9:FALSE ("enabled"), 11:w81) -> ()  [unwired: 1 in, 5 out]
        n62 = local write "Sync"(w65) -> ()
        n63 = call <resource>:"UMLEditor_GraphMemory.vi"("GraphIn"=w83) -> ()  [unwired: 1 in, 18 out]
        n64 = Bundle By Name(cluster=w114, "Sync"=w65, "ToolHelp"=w97, "menu"=w81, "grid"=w145, "graphics"=w143, "toolType"=UMLEditor_tooltype."None", "tool"=UMLEditor_toolsType."CD_Select", "diagramIndex"=0, "zoom"=1.0, "hideGrid"=FALSE, "lastMousePoint"=w137, "rubberBandStart"=w137, "dragStartPoint"=w137, "dragStartBounds"=T13 {"x"=nan, "y"=nan, "width"=nan, "height"=nan}, "gridColor"=w76, "gridSize"=w75, "CONNECT_THRESHOLD"=8, "selcted"=UMLEditor_tooltype."None", "diagrams"=w130, "offset"=T12 {"x"=0.0, "y"=0.0}, "Event"=w85, "file"=w68, "SyncTime"=w66) -> (w94:T7)
        n65 = call <resource>:"UMLEditor menuUpdates.vi"("menu"=w81, "menuAction"=UMLEditor_MenuActionType."DiableSave", "error in (no error)"=w92) -> ("error out"=w116:errorcluster)  [unwired: 3 in, 13 out]
        n66 = property on="Picture" class="Pict"("Origin:Left"=w111, "Origin:Top"=w111) -> ()  [unwired: 2 in, 2 out]
        n67 = property on="toolTab" class="TabCtl (strict)"("Disabled"=u8 0) -> ()  [unwired: 2 in, 2 out]
        n68 = call <resource>:"UMLEditor updateDiagramsInfo.vi"("localVariables"=w94, "error in (no error)"=w116) -> ("diagramNames"=w122:string[], "index"=w121:i32, "error out"=w112:errorcluster)  [unwired: 15 out]
        n69 = local write "Diagram"(w121) -> ()
        n70 = property on="Diagram" class="Ring (strict)"("Strings []"=w122) -> ()  [unwired: 2 in, 2 out]
      }
      frame "Init2" {
        n71 = call <resource>:"GDSProject_GetProjects.vi"("error in (no error)"=w202, "OpenProjectRef(True)"=FALSE) -> ("Projects"=w198:string[], "error out"=w200:errorcluster)  [unwired: 1 in, 15 out]
        n72 = local write "StatusBar"("" ("StatusBar")) -> ()
        n73 = Empty String/Path?(string/path=w174) -> (empty?=w176:bool)
        n74 = Search 1D Array(1D array=w198, element=w195) -> (index of element=w197:i32)  [unwired: 1 out]
        n75 = call <resource>:"File_ApplicationPaths.vi"("PathName"=UMLEditor_StoredPathes."WizDir" ("UMLPathes")) -> ()  [unwired: 3 in, 16 out]
        n76 = case shown="0, Default" w197 {
          selector: w197 -> [w216 _]
          tunnel: [w216 u8 0 ("t")] -> w196
          frame 0, Default {
          }
          frame -1 {
          }
        }
        n77 = Select(t="My Computer" ("element"), s=w176, f=w174) -> (s? t:f=w173:string)
        n78 = Index Array(array=w198, index=w196) -> (element=w201:string)
        n79 = Empty Array?(array=w198) -> (empty?=w199:bool)
        n80 = property on="Project" class="Ring (strict)"("Strings []"=w198, "Value"=w196) -> ()  [unwired: 2 in, 2 out]
        n81 = case shown="False" w199 {
          tunnel: w201 -> [w226 _]
          tunnel: w200 -> [w225 w230]
          tunnel: [w224 w230] -> w193
          tunnel: [w223 _] -> w178
          tunnel: [w222 _] -> w177
          tunnel: w173 -> [w221 _]
          frame False {
            n82 = call <resource>:"UMLEditor_TargetDialog.vi"("error in (no error)"=w225, "Target"=w221, "GetProjectRefByName"=w226) -> ("error out"=w224:errorcluster, "ProjectFolder"=w218:path, "TargetIndex"=w222:u16, "Targets"=w223:string[])  [unwired: 4 in, 1 out]
            n83 = call <resource>:"GetRelativePathOption.vi"() -> ("UseProjectFolderAsBasePath"=w220:bool)  [unwired: 1 in, 18 out]
            n84 = case shown="True" w220 {
              tunnel: w218 -> [_ w228]
              tunnel: File_StoredPathesActions."Set Path" ("Method (Get Path)") -> [_ w227]
              frame False {
              }
              frame True {
                n85 = call <resource>:"File_ApplicationPaths.vi"("PathName"=UMLEditor_StoredPathes."ClassBasePath" ("UMLPathes"), "Path In"=w228, "Method (Get Path)"=w227) -> ()  [unwired: 1 in, 16 out]
              }
            }
          }
          frame True {
          }
        }
        n86 = property on="Target" class="Ring (strict)"("Strings []"=w178, "Value"=w177) -> ()  [unwired: 2 in, 2 out]
        n87 = Unbundle By Name(w183) -> ("menu"=w186:refnum<k9>)
        n88 = call <resource>:"UMLEditor ControlBusyDialog.vi"("error in (no error)"=w193, "Action(SendStatusMessage)"=UMLEditor_BusyDialogAction."Initialize" ("Action")) -> ("error out"=w204:errorcluster)  [unwired: 2 in, 15 out]
        n89 = call <resource>:"GetToolTip.vi"("error in (no error)"=w193) -> ("ToolTip"=w192:cluster{"ToolTipOpen":bool, "LastToolTip":i32})  [unwired: 18 out]
        n90 = call <resource>:"UMLEditor AddToolsMenuItems.vi"("menu"=w186, "GoopWizExists"=FALSE, "error in (no error)"=w204) -> ("error out"=w212:errorcluster)  [unwired: 1 in, 15 out]
        n91 = Unbundle By Name(w192) -> ("ToolTipOpen"=w191:bool)
        n92 = Current VI's Path() -> (path=w211:path)
        n93 = Open VI Reference(vi path=w211, error in (no error)=w212) -> (vi reference=w206:refnum<vi>, error out=w213:errorcluster)  [unwired: 4 out]
        n94 = Unbundle By Name(w183) -> ("ToolHelp"=w208:bool)
        n95 = case shown="False" w191 {
          frame False {
          }
          frame True {
            n96 = call <resource>:"ShowToolTips.vi"() -> ()  [unwired: 1 in, 19 out]
          }
        }
        n97 = call <resource>:"ContextHelp_StartPopUpTask.vi"("CallerRef"=w206, "error in (no error)"=w213) -> ("PopUpTaskEvent"=w205:T17, "error out"=w209:errorcluster)  [unwired: 16 out]
        n98 = call <resource>:"ContextHelp_Memory.vi"("State"=w208, "error in (no error)"=w209, "Actio(GetStatus)n"=T27."SetToolHelp") -> ("error out"=w185:errorcluster)  [unwired: 1 in, 15 out]
        n99 = call <resource>:"UMLEditor menuUpdates.vi"("menu"=w186, "menuAction"=UMLEditor_MenuActionType."disablePropDel") -> ()  [unwired: 4 in, 14 out]
        n100 = Bundle By Name(cluster=w183, "ViRef"=w206, "PopUpMessageEvent"=w205) -> (w207:T7)
        n101 = call <resource>:"UMLEditor getDiagramInfo.vi"("localVariables"=w183, "error in (no error)"=w185) -> ("graph"=w184:refnum<class "Graph.lvclass">, "error out"=w182:errorcluster)  [unwired: 16 out]
        n102 = call <resource>:"GetUndoOption.vi"("error in (no error)"=w182) -> ("UndoSize"=w180:i32, "error out"=w181:errorcluster)  [unwired: 17 out]
        n103 = call <resource>:"UndoEngine.vi"("reference"=w184, "Action"=enum16{"TakeSnapshot", "Undo", "Redo"}."TakeSnapshot", "Reset"=TRUE, "error in (no error)"=w181, "menu"=w186, "UndoLevels(ignoredIfNotWired)"=w180) -> ("error out"=w187:errorcluster)  [unwired: 2 in, 11 out]
      }
      frame "Init3" {
        (unwired) UMLEditor_Cursortype."NWSE" ("CursorType")
        n104 = call <resource>:"GOOP_GetGDSConfigFolder.vi"() -> ("GDSFolderPath"=w242:path)
        n105 = Build Path(base path=w242, name or relative path="Cursors") -> (appended path=w239:path)
        n106 = Create Folder(path (use dialog)=w239) -> (created path=w238:path, error out=w237:errorcluster)  [unwired: 2 in, 1 out]
        n107 = for {
          tunnel: w239 -> [w261]
          tunnel: string[] ["ns", "we", "nesw", "nwse"] -> [w257] mode=indexing
          shift-right: [w248] -> w245
          shift-left: w246 -> [w251]
          tunnel: [w258] -> w243 mode=indexing
          tunnel: string[] ["\u0000\u0000\u0002\u0000\u0001\u0000  \u0000\u0000\u000f\u0000\u0010\u00000\u0001\u0000\u0000\u0016\u0000\u0000\u0000(\u0000\u0000\u0000 \u0000\u0000\u0000@\u0000\u0000\u0000\u0001\u0000\u0001\u0000\u0000\u0000\u0000\u0000\u0000\u0001\u0000\u0000\u0000\u0000\u0000\u0000\u0000\u0000\u0000\u0000\u0000\u0000\u0000\u0000\u0000\u0000\u0000\u0000\u0000\u0000\u0000\u0000ÿÿÿ\u0000\u0000\u0000\u0000\u0000\u0000\u0000\u0000\u0000\u0000\u0000\u0000\u0000\u0000\u0000\u0000\u0000\u0000\u0000\u0000\u0000\u0000\u0001\u0000\u0000\u0000\u0002€\u0000\u0000\u0004@\u0000\u0000\b \u0000\u0000\u0010\u0010\u0000\u0000\u001eð\u0000\u0000\u0002€\u0000\u0000\u0002€\u0000\u0000\u0002€\u0000\u0000\u0002€\u0000\u0000\u0002€\u0000\u0000\u0002€\u0000\u0000\u0002€\u0000\u0000\u0002€\u0000\u0000\u001eð\u0000\u0000\u0010\u0010\u0000\u0000\b \u0000\u0000\u0004@\u0000\u0000\u0002€\u0000\u0000\u0001\u0000\u0000\u0000\u0000\u0000\u0000\u0000\u0000\u0000\u0000\u0000\u0000\u0000\u0000\u0000\u0000\u0000\u0000\u0000\u0000\u0000\u0000\u0000\u0000\u0000\u0000\u0000\u0000\u0000\u0000ÿÿÿÿÿÿÿÿÿÿÿÿÿÿÿÿÿÿÿÿÿþÿÿÿüÿÿø?ÿÿð\u001fÿÿà\u000fÿÿà\u000fÿÿüÿÿüÿÿüÿÿüÿÿüÿÿüÿÿüÿÿüÿÿà\u000fÿÿà\u000fÿÿð\u001fÿÿø?ÿÿüÿÿþÿÿÿÿÿÿÿÿÿÿÿÿÿÿÿÿÿÿÿÿÿÿÿÿÿÿÿÿÿÿ", "\u0000\u0000\u0002\u0000\u0001\u0000  \u0000\u0000\u0010\u0000\u0010\u00000\u0001\u0000\u0000\u0016\u0000\u0000\u0000(\u0000\u0000\u0000 \u0000\u0000\u0000@\u0000\u0000\u0000\u0001\u0000\u0001\u0000\u0000\u0000\u0000\u0000\u0000\u0001\u0000\u0000\u0000\u0000\u0000\u0000\u0000\u0000\u0000\u0000\u0000\u0000\u0000\u0000\u0000\u0000\u0000\u0000\u0000\u0000\u0000\u0000ÿÿÿ\u0000\u0000\u0000\u0000\u0000\u0000\u0000\u0000\u0000\u0000\u0000\u0000\u0000\u0000\u0000\u0000\u0000\u0000\u0000\u0000\u0000\u0000\u0000\u0000\u0000\u0000\u0000\u0000\u0000\u0000\u0000\u0000\u0000\u0000\u0000\u0000\u0000\u0000\u0000\u0000\u0000\u0000\u0000\u0000\u0000\u00000\u0006\u0000\u0000P\u0005\u0000\u0000\u0004\u0001\u001fü@\u0002\u0000\u0000 \u0001\u001fü@\u0000\u0004\u0000P\u0005\u0000\u00000\u0006\u0000\u0000\u0000\u0000\u0000\u0000\u0000\u0000\u0000\u0000\u0000\u0000\u0000\u0000\u0000\u0000\u0000\u0000\u0000\u0000\u0000\u0000\u0000\u0000\u0000\u0000\u0000\u0000\u0000\u0000\u0000\u0000\u0000\u0000\u0000\u0000\u0000\u0000\u0000\u0000\u0000\u0000\u0000\u0000\u0000\u0000\u0000\u0000\u0000ÿÿÿÿÿÿÿÿÿÿÿÿÿÿÿÿÿÿÿÿÿÿÿÿÿÿÿÿÿÿÿÿÿÿÿÿÿÿÿÿÿÿÿÿÿÏùÿÿøÿÿ\u000føþ\u0000\u0000?ü\u0000\u0000\u001fþ\u0000\u0000?ÿ\u000føÿøÿÿÏùÿÿÿÿÿÿÿÿÿÿÿÿÿÿÿÿÿÿÿÿÿÿÿÿÿÿÿÿÿÿÿÿÿÿÿÿÿÿÿÿÿÿÿÿÿÿÿÿÿ", "\u0000\u0000\u0002\u0000\u0001\u0000  \u0000\u0000\u0010\u0000\u0010\u00000\u0001\u0000\u0000\u0016\u0000\u0000\u0000(\u0000\u0000\u0000 \u0000\u0000\u0000@\u0000\u0000\u0000\u0001\u0000\u0001\u0000\u0000\u0000\u0000\u0000\u0000\u0001\u0000\u0000\u0000\u0000\u0000\u0000\u0000\u0000\u0000\u0000\u0000\u0000\u0000\u0000\u0000\u0000\u0000\u0000\u0000\u0000\u0000\u0000ÿÿÿ\u0000\u0000\u0000\u0000\u0000\u0000\u0000\u0000\u0000\u0000\u0000\u0000\u0000\u0000\u0000\u0000\u0000\u0000\u0000\u0000\u0000\u0000\u0000\u0000\u0000\u0000\u0000\u0000\u0000\u0000\u0000\u0000\u0000\u0000\u0000\u0000\u0000A\u0000\u0000\u0000B\u0000\u0000\u0000D\u0000\u0000\u0000J\u0000\u0000\u0000U\u0000\u0000\u0000b\u0000\u0000\u0001@\u0000\u0000\u0000£\u0000\u0000\u0000U\u0000\u0000\u0000)\u0000\u0000\u0000\u0011\u0000\u0000\u0000!\u0000\u0000\u0000A\u0000\u0000\u0000\u0000\u0000\u0000\u0000\u0000\u0000\u0000\u0000\u0000\u0000\u0000\u0000\u0000\u0000\u0000\u0000\u0000\u0000\u0000\u0000\u0000\u0000\u0000\u0000\u0000\u0000\u0000\u0000\u0000\u0000\u0000\u0000\u0000\u0000\u0000\u0000\u0000ÿÿÿÿÿÿÿÿÿÿÿÿÿÿÿÿÿÿÿÿÿÿÿÿÿÿÿÿÿÿÿÿÿÿÿÿÿÿÿÿÿÿÿÿÿÿÿÿÿÿÿÿÿþ?ÿÿÿ\u001cÿÿÿÿÿÿÀÿÿÿàÿÿÿÀÿÿÿÿÿÿÿÿÿÿÿÿÿÿÿÿÿÿÿÿÿÿÿÿÿÿÿÿÿÿÿÿÿÿÿÿÿÿÿÿÿÿÿ", "\u0000\u0000\u0002\u0000\u0001\u0000  \u0000\u0000\u0010\u0000\u0010\u00000\u0001\u0000\u0000\u0016\u0000\u0000\u0000(\u0000\u0000\u0000 \u0000\u0000\u0000@\u0000\u0000\u0000\u0001\u0000\u0001\u0000\u0000\u0000\u0000\u0000\u0000\u0001\u0000\u0000\u0000\u0000\u0000\u0000\u0000\u0000\u0000\u0000\u0000\u0000\u0000\u0000\u0000\u0000\u0000\u0000\u0000\u0000\u0000\u0000ÿÿÿ\u0000\u0000\u0000\u0000\u0000\u0000\u0000\u0000\u0000\u0000\u0000\u0000\u0000\u0000\u0000\u0000\u0000\u0000\u0000\u0000\u0000\u0000\u0000\u0000\u0000\u0000\u0000\u0000\u0000\u0000\u0000\u0000\u0000\u0000\u0000\u0000\u0000\u0000A\u0000\u0000\u0000!\u0000\u0000\u0000\u0011\u0000\u0000\u0000)\u0000\u0000\u0000U\u0000\u0000\u0000£\u0000\u0000\u0001@\u0000\u0000b\u0000\u0000U\u0000\u0000\u0000J\u0000\u0000\u0000D\u0000\u0000\u0000B\u0000\u0000\u0000A\u0000\u0000\u0000\u0000\u0000\u0000\u0000\u0000\u0000\u0000\u0000\u0000\u0000\u0000\u0000\u0000\u0000\u0000\u0000\u0000\u0000\u0000\u0000\u0000\u0000\u0000\u0000\u0000\u0000\u0000\u0000\u0000\u0000\u0000\u0000\u0000\u0000\u0000\u0000\u0000\u0000ÿÿÿÿÿÿÿÿÿÿÿÿÿÿÿÿÿÿÿÿÿÿÿÿÿÿÿÿÿÿÿÿÿÿÿÿÿÿÿÿÀÿÿÿàÿÿÿÀÿÿÿÿÿÿ\u001cÿÿþ?ÿÿÿÿÿÿÿÿÿÿÿÿÿÿÿÿÿÿÿÿÿÿÿÿÿÿÿÿÿÿÿÿÿÿÿÿÿÿÿÿÿÿÿÿÿÿÿÿÿÿÿÿÿÿÿÿÿ"] -> [w249] mode=indexing
          tunnel: w238 -> [_]
          tunnel: w237 -> [_]
          i -> [w260]
          n108 = Concatenate Strings(w257, "1.cur" ("string")) -> (w255:string)
          n109 = Build Path(base path=w261, name or relative path=w255) -> (appended path=w253:path)
          n110 = call <vilib>:"Check if File or Folder Exists.vi"("path"=w253) -> ("file or folder exists?"=w252:bool, "dup path"=w250:path)  [unwired: 8 in, 1 out]
          n111 = case shown="False" w252 {
            tunnel: w251 -> [w265 w266]
            tunnel: [w264 w266] -> w248
            tunnel: w250 -> [w263 _]
            tunnel: w249 -> [w262 _]
            frame False {
              n112 = Write to Text File(file (use dialog)=w263, text=w262, error in=w265) -> (error out=w264:errorcluster)  [unwired: 1 in, 2 out]
            }
            frame True {
            }
          }
          n113 = Add(x=i16 20 ("cursor resource ID"), y=w260) -> (x+y=w254:i32)
          n114 = call <vilib>:"Create Cursor From File.vi"("error in (no error)"=w248, "cursor resource ID"=w254, "cursor file"=w250) -> ("cursor ID"=w258:refnum<k1>)  [unwired: 1 in, 7 out]
        }
        n115 = Unbundle By Name(w236) -> ("file"=w235:path)
        n116 = Empty String/Path?(string/path=w235) -> (empty?=w234:bool)
        n117 = Bundle By Name(cluster=w236, "Cursors"=w243) -> (w244:T7)
        n118 = Select(t=UMLEditor_statesType."Idle" ("state"), s=w234, f=UMLEditor_statesType."Open" ("state")) -> (s? t:f=w231:T8)
      }
      frame "Idle" {
        n119 = Unbundle By Name(w272) -> ("butDwn"=w283:bool, "Event"=w273:refnum<event-registration>)
        n120 = Bundle By Name(cluster=w272, "state"=w276) -> (w277:T7)
